vi "CommandDSA.vi"(4 "error in (no error)":errorcluster, 5 "timeout ms (20000)":i32=20000, 6 "command":string, 7 "connection ID":refnum<k5>) -> (0 "error out":errorcluster, 1 "bytes read":i32, 2 "data out":string, 3 "connection ID out":refnum<k5>)   [LabVIEW 2019]
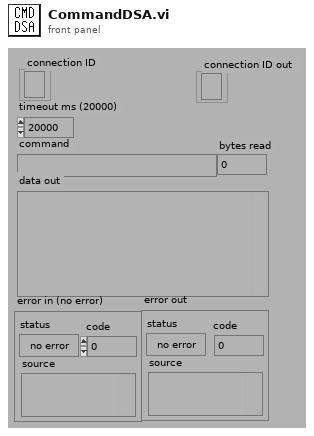
[diagram p1: front panel]
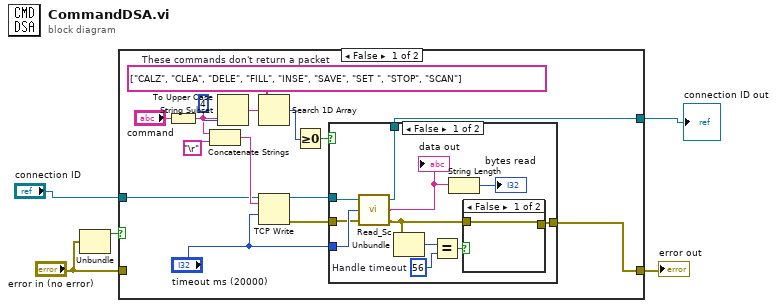
[diagram p0: block diagram]
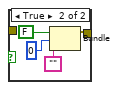
[diagram p2: hidden frame]
diagram:
  n1 = Unbundle("error in (no error)") -> ("status"=w3:bool)  [unwired: 2 out]
  n2 = case shown="False" w3 {
    tunnel: [w8 w40] -> w4
    tunnel: "error in (no error)" -> [_ w40]
    tunnel: "connection ID" -> [w7 w39]
    tunnel: [w6 w39] -> w1
    frame False {
      w10 = string[] ["CALZ", "CLEA", "DELE", "FILL", "INSE", "SAVE", "SET ", "STOP", "SCAN"]  # These commands don't return a packet
      n3 = To Upper Case(1:"command") -> (0:w11:string)
      n4 = Concatenate Strings(w11, "\r") -> (w20:string)
      n5 = String Subset(string=w11, length (rest)=4) -> (substring=w16:string)  [unwired: 1 in]
      n6 = Search 1D Array(1D array=w10, element=w16) -> (index of element=w15:i32)  [unwired: 1 in]
      n7 = TCP Write(connection ID=w7, data in=w20, 9:"timeout ms (20000)") -> (connection ID out=w19:refnum<k5>, error out=w18:errorcluster)  [unwired: 1 in, 1 out]
      n8 = Greater Or Equal To 0?(x=w15) -> (x >= 0?=w14:bool)
      n9 = case shown="False" w14 {
        tunnel: [w30 w38] -> w8
        tunnel: w18 -> [w21 w38]
        tunnel: w19 -> [w23 w37]
        tunnel: "timeout ms (20000)" -> [w22 _]
        tunnel: [w24 w37] -> w6
        frame False {
          w28 = 56  # Handle timeout
          n10 = call "Read_Sc.vi"("error in (no error)"=w21, "timeout ms (10000)"=w22, "connection ID"=w23) -> ("error out"=w26:errorcluster, "data out"=w25:string, "connection ID out"=w24:refnum<k5>)
          "data out" <- w25
          n11 = Unbundle(w26) -> ("code"=w29:i32)  [unwired: 2 out]
          n12 = Equal?(x=w29, y=w28) -> (x = y?=w31:bool)
          n13 = String Length(string=w25) -> (length=→"bytes read":i32)
          n14 = case shown="False" w31 {
            tunnel: [w32 w33] -> w30
            tunnel: w26 -> [w32 _]
            frame False {
            }
            frame True {
              n15 = Bundle(FALSE, 0, "") -> (w33:errorcluster)  [unwired: 1 in]
            }
          }
        }
        frame True {
        }
      }
    }
    frame True {
      (unwired) ""
      (unwired) 0
    }
  }
  "error out" <- w4
  "connection ID out" <- w1
